vi "Pre Launch Init.vi"(11 "Device in":refnum<class "Device.lvclass">) -> (0 "error out":errorcluster, 3 "Device out":refnum<class "Device.lvclass">)   [LabVIEW 2020, in "Device.lvlib" / "Device.lvclass"]
doc: "(<B>Filename</B>: Actor Framework.lvlib:Actor.lvclass:Pre Launch Init.vi)\n\nDefines behavior that occurs after the Launch Nested Actor method is invoked but before the actor's Actor Core method begins running.\n\nBy default, this method does nothing. A descendant class may override it to define behavior."
uses:
  Device.lvclass
  <vilib>/ActorFramework/Actor/Actor.lvclass
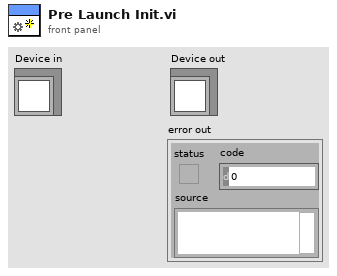
[diagram p1: front panel]
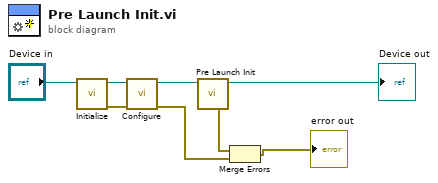
[diagram p0: block diagram]
diagram:
  n1 = call-dynamic "Initialize.vi"("Device in"="Device in") -> ("error out"=w4:errorcluster, "Device out"=w6:refnum<class "Device.lvclass">)  [unwired: 9 in]
  n2 = call-dynamic "Configure.vi"("error in (no error)"=w4, "Device in"=w6) -> ("error out"=w1:errorcluster, "Device out"=w5:refnum<class "Device.lvclass">)  [unwired: 8 in]
  n3 = call-parent "Pre Launch Init.vi"("Actor in"=w5) -> ("error out"=w2:errorcluster, "Actor out"=→"Device out":refnum<class "Device.lvclass">)  [unwired: 9 in]
  n4 = Merge Errors(w2, w1) -> (→"error out":errorcluster)
